vi "Open caller's caller.vi"(5 "error in (no error)":errorcluster, 8 "vi reference":refnum<vi>) -> (0 "error out":errorcluster)   [LabVIEW 2016]
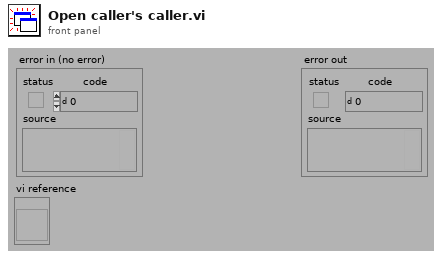
[diagram p1: front panel]
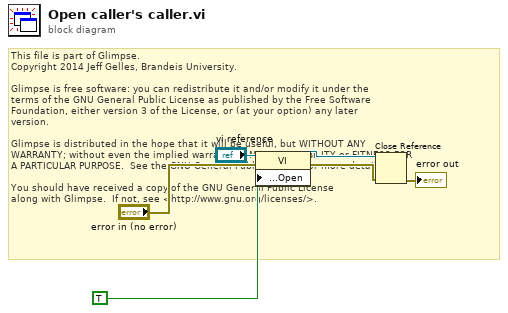
[diagram p0: block diagram]
diagram:
  # "This file is part of Glimpse. \nCopyright 2014 Jeff Gelles, Brandeis University.    \n\nGlimpse is free software: you can redistribute it and/or modify it under the \nterms of the GNU General Public License as published by the Free Software \nFoundation, either version 3 of the License, or (at your option) any later \nversion.\n\nGlimpse is distributed in the hope that it will be useful, but WITHOUT ANY \nWARRANTY; without even the implied warranty of MERCHANTABILITY or FITNESS FOR \nA PARTICULAR PURPOSE.  See the GNU General Public License for more details.\n\nYou should have received a copy of the GNU General Public License\nalong with Glimpse.  If not, see <http://www.gnu.org/licenses/>."
  n1 = property class="VI"(reference="vi reference", error in="error in (no error)", "Front Panel Window:Open"=TRUE) -> (reference out=w2:refnum<vi>, error out=w1:errorcluster)
  n2 = Close Reference(reference=w2, error in (no error)=w1) -> (error out=→"error out":errorcluster)
